vi "Initial Values-format and values-Live window.vi"() -> (13 "Values.Boolean":bool[](array[boolean]), 14 "Keys setup.DBL":T2=[{"key"="Control FPGA.Clock Freq (MHz)", "Save?"=TRUE, "Default"=240.0}, {"key"="DAQ FPGA.Clock Freq (MHz)", "Save?"=TRUE, "Default"=240.0}], 15 "Values.DBL":dbl[](array[numeric]), 16 "Keys setup.String":T3=[{"key"="Control FPGA.MAC address", "Save?"=TRUE, "Default"="AABBCCDDEEFF"}, {"key"="DAQ FPGA.Target", "Save?"=TRUE, "Default"="RIO0"}, {"key"="XY Stage.COM port", "Save?"=TRUE, "Default"="COM7"}, {"key"="DAQmx Chan.Pockels Control", "Save?"=TRUE, "Default"=""}, {"key"="DAQmx Chan.Hard Shutter", "Save?"=TRUE, "Default"=""}, {"key"="DAQmx Chan.PMT 1", "Save?"=TRUE, "Default"=""}, {"key"="DAQmx Chan.PMT 2", "Save?"=TRUE, "Default"=""}, {"key"="DAQmx Chan.Encoder Trigger", "Save?"=TRUE, "Default"=""}, {"key"="DAQmx Chan.Optional Trigger 1", "Save?"=TRUE, "Default"=""}, {"key"="DAQmx Chan.Optional Trigger 2", "Save?"=TRUE, "Default"=""}, {"key"="DAQmx Chan.Optional Trigger 3", "Save?"=TRUE, "Default"=""}], 17 "Values.Strings":string[](array[string]), 18 "Keys setup.Boolean":T1, 19 "error out":errorcluster)   [LabVIEW 2017]
uses:
  Typedefs/Ini file interface (String).ctl
  Typedefs/Ini file interface (DBL).ctl
  Typedefs/Ini file interface (Boolean).ctl
  User Interface/Globals/gl_Windows Ctrl refs.vi
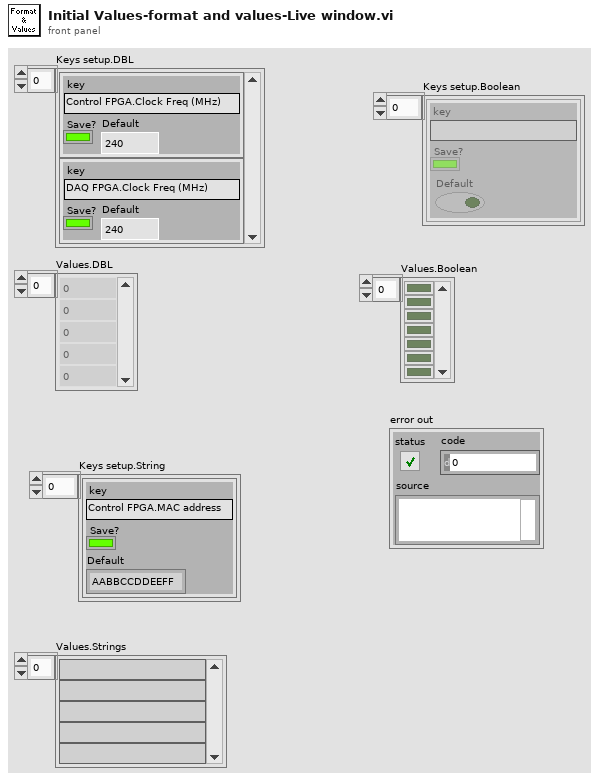
[diagram p1: front panel]
types:
  T1 = typedef "Ini file interface (Boolean).ctl" = cluster{"key":string, "Save?":bool, "Default":bool}[]
  T2 = typedef "Ini file interface (DBL).ctl" = cluster{"key":string, "Save?":bool, "Default":dbl}[]
  T3 = typedef "Ini file interface (String).ctl" = cluster{"key":string, "Save?":bool, "Default":string}[]
  T4 = typedef "Live window-ctrl refs.ctl" = cluster{"This VI":refnum<vi>, "Pane":refnum<vi>, "Snapshot":refnum<vi>, "Left Image Palette":refnum<vi>, "Right Image Palette":refnum<vi>, "Left Channel":refnum<vi>, "Right Channel":refnum<vi>, "Left image intensity":refnum<vi>, "Right image intensity":refnum<vi>, "Left Image Display":T5, "Right Image Display":T5, "Refresh rate ind (Hz)":refnum<vi>, "Acq rate ind (Hz)":refnum<vi>, "Stop (ind)":refnum<vi>}
  T5 = typedef "Image display ref.ctl" = refnum<vi>
  T6 = typedef "Channel Selector.ctl" = enum16{"Red Channel", "Green Channel", "Blended"}
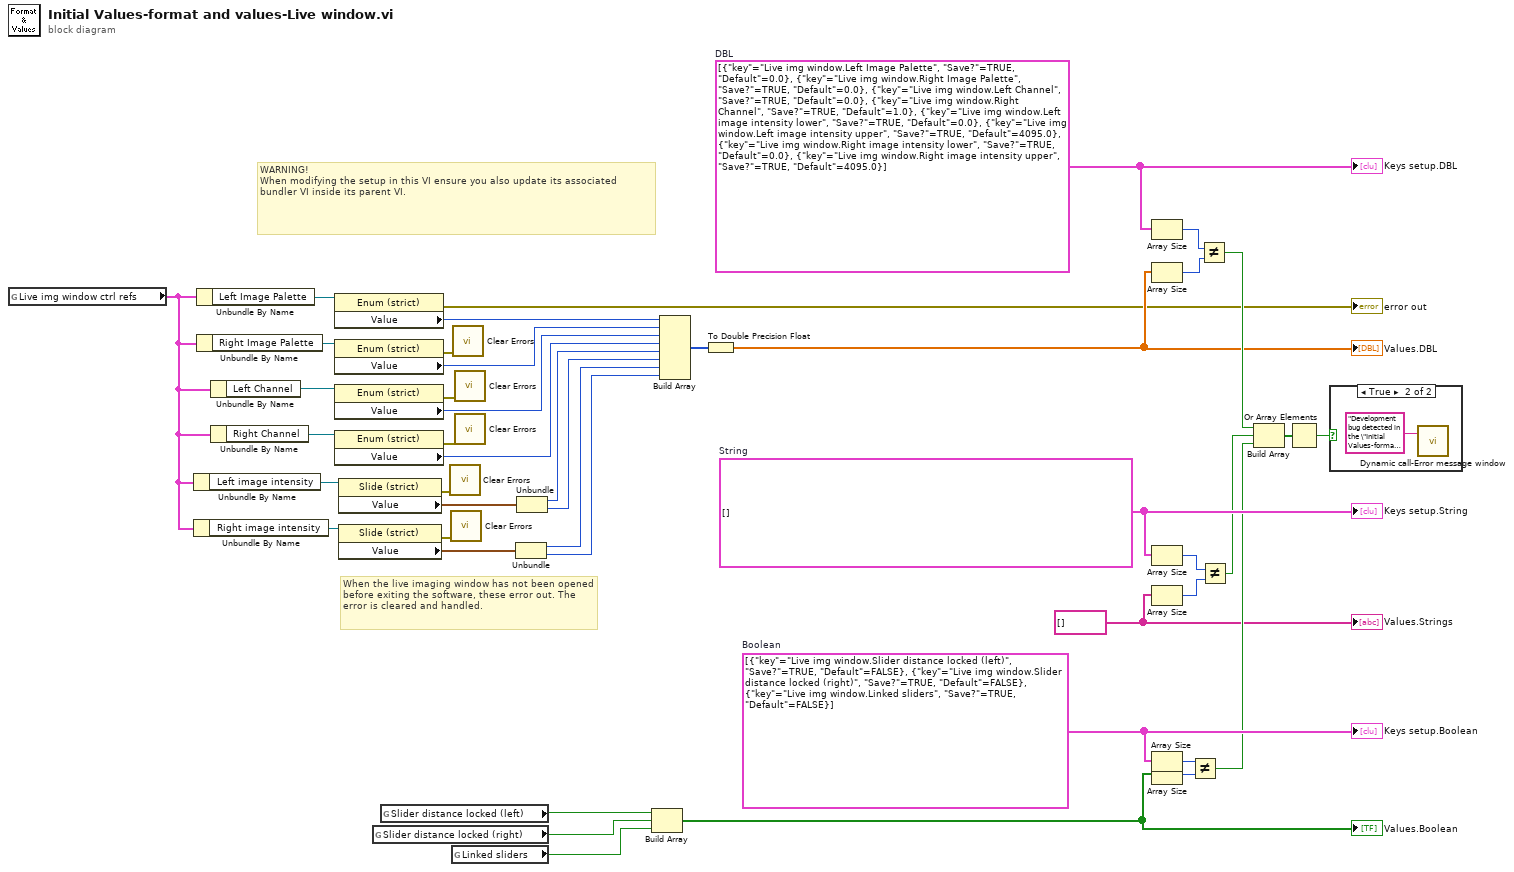
[diagram p0: block diagram]
diagram:
  w28 = string[] [] ("appended array")
  w41 = T1 [{"key"="Live img window.Slider distance locked (left)", "Save?"=TRUE, "Default"=FALSE}, {"key"="Live img window.Slider distance locked (right)", "Save?"=TRUE, "Default"=FALSE}, {"key"="Live img window.Linked sliders", "Save?"=TRUE, "Default"=FALSE}]  # Boolean
  w44 = T3 []  # String
  w43 = T2 [{"key"="Live img window.Left Image Palette", "Save?"=TRUE, "Default"=0.0}, {"key"="Live img window.Right Image Palette", "Save?"=TRUE, "Default"=0.0}, {"key"="Live img window.Left Channel", "Save?"=TRUE, "Default"=0.0}, {"key"="Live img window.Right Channel", "Save?"=TRUE, "Default"=1.0}, {"key"="Live img window.Left image intensity lower", "Save?"=TRUE, "Default"=0.0}, {"key"="Live img window.Left image intensity upper", "Save?"=TRUE, "Default"=4095.0}, {"key"="Live img window.Right image intensity lower", "Save?"=TRUE, "Default"=0.0}, {"key"="Live img window.Right image intensity upper", "Save?"=TRUE, "Default"=4095.0}]  # DBL
  # "When the live imaging window has not been opened before exiting the software, these error out. The error is cleared and handled."
  # "WARNING!\nWhen modifying the setup in this VI ensure you also update its associated bundler VI inside its parent VI."
  n1 = global read "gl_Windows Ctrl refs.vi" "Live img window ctrl refs"() -> (w1:T4)
  n2 = Unbundle By Name(w1) -> ("Left image intensity"=w18:refnum<vi>)
  n3 = Unbundle By Name(w1) -> ("Right image intensity"=w19:refnum<vi>)
  n4 = Unbundle By Name(w1) -> ("Left Image Palette"=w29:refnum<vi>)
  n5 = Unbundle By Name(w1) -> ("Right Image Palette"=w26:refnum<vi>)
  n6 = Unbundle By Name(w1) -> ("Left Channel"=w23:refnum<vi>)
  n7 = Unbundle By Name(w1) -> ("Right Channel"=w24:refnum<vi>)
  n8 = property class="Enum (strict)"(reference=w29) -> (error out=→"error out":errorcluster, "Value"=w27:enum16{"Gray", "Red", "Green"})  [unwired: 1 in, 1 out]
  n9 = property class="Enum (strict)"(reference=w26) -> (error out=w11:errorcluster, "Value"=w25:enum16{"Gray", "Red", "Green"})  [unwired: 1 in, 1 out]
  n10 = property class="Enum (strict)"(reference=w23) -> (error out=w10:errorcluster, "Value"=w22:T6)  [unwired: 1 in, 1 out]
  n11 = property class="Enum (strict)"(reference=w24) -> (error out=w9:errorcluster, "Value"=w21:T6)  [unwired: 1 in, 1 out]
  n12 = property class="Slide (strict)"(reference=w18) -> (error out=w8:errorcluster, "Value"=w17:cluster{i16, i16})  [unwired: 1 in, 1 out]
  n13 = property class="Slide (strict)"(reference=w19) -> (error out=w7:errorcluster, "Value"=w16:cluster{i16, i16})  [unwired: 1 in, 1 out]
  n14 = global read "gl_Windows Ctrl refs.vi" "Slider distance locked (right)"() -> (w4:bool)
  n15 = global read "gl_Windows Ctrl refs.vi" "Slider distance locked (left)"() -> (w5:bool)
  n16 = call <vilib>:"Clear Errors.vi"("error in (no error)"=w8) -> ()  [unwired: 5 in, 2 out]
  n17 = call <vilib>:"Clear Errors.vi"("error in (no error)"=w7) -> ()  [unwired: 5 in, 2 out]
  n18 = global read "gl_Windows Ctrl refs.vi" "Linked sliders"() -> (w2:bool)
  n19 = call <vilib>:"Clear Errors.vi"("error in (no error)"=w11) -> ()  [unwired: 5 in, 2 out]
  n20 = call <vilib>:"Clear Errors.vi"("error in (no error)"=w10) -> ()  [unwired: 5 in, 2 out]
  n21 = call <vilib>:"Clear Errors.vi"("error in (no error)"=w9) -> ()  [unwired: 5 in, 2 out]
  n22 = Unbundle(w16) -> (w13:i16, w12:i16)
  n23 = Unbundle(w17) -> (w15:i16, w14:i16)
  n24 = Build Array(w5, w4, w2) -> (w3:bool[])
  "Values.Boolean" <- w3
  n25 = Build Array(w27, w25, w22, w21, w15, w14, w13, w12) -> (w42:u16[])
  n26 = To Double Precision Float(number=w42) -> (double precision float=w20:dbl[])
  "Values.DBL" <- w20
  n27 = Array Size(array=w43) -> (size(s)=w38:i32)
  n28 = Array Size(array=w20) -> (size(s)=w37:i32)
  n29 = Array Size(array=w44) -> (size(s)=w40:i32)
  n30 = Array Size(array=w28) -> (size(s)=w39:i32)
  n31 = Array Size(array=w41) -> (size(s)=w36:i32)
  n32 = Array Size(array=w3) -> (size(s)=w35:i32)
  n33 = Not Equal?(x=w36, y=w35) -> (x != y?=w33:bool)
  n34 = Not Equal?(x=w38, y=w37) -> (x != y?=w31:bool)
  n35 = Not Equal?(x=w40, y=w39) -> (x != y?=w30:bool)
  n36 = Build Array(w31, w30, w33) -> (w34:bool[])
  n37 = Or Array Elements(Boolean array=w34) -> (logical OR=w32:bool)
  n38 = case shown="True" w32 {
    frame False {
    }
    frame True {
      n39 = call "Dynamic call-Error message window.vi"("Error Message"="Development bug detected in the \"Initial Values-format and values-Live window.vi\".\nPlease correct the set up in this VI.") -> ()  [unwired: 10 in, 1 out]
    }
  }
  "Keys setup.String" <- w44
  "Keys setup.DBL" <- w43
  "Values.Strings" <- w28
  "Keys setup.Boolean" <- w41
